vi "Create Data Table.vi"(8 "错误输入（无错误）":errorcluster, 9 "Result":bool[](array[boolean]), 10 "Data":bool[][](array[boolean]), 11 "Data Table":refnum<vi>) -> (0 "错误输出":errorcluster, 3 "Data Table Ref Out":refnum<vi>)   [LabVIEW 2012]
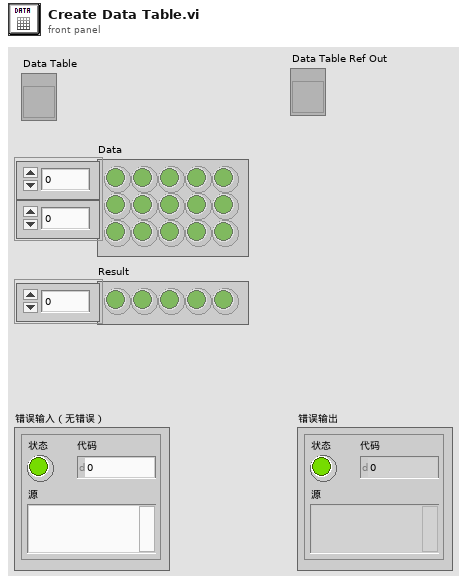
[diagram p1: front panel]
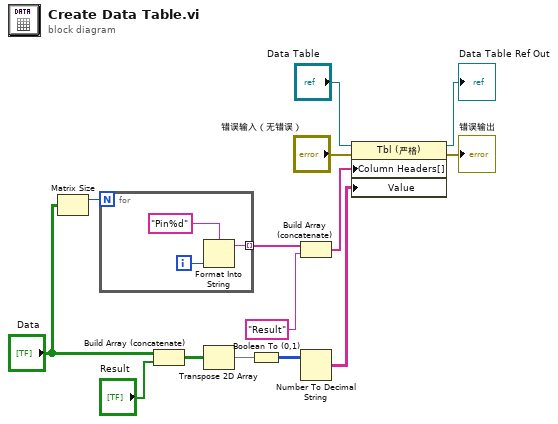
[diagram p0: block diagram]
diagram:
  n1 = Matrix Size(0:"Data") -> (1:w14:i32)  [unwired: 1 out]
  n2 = for {
    N: w14 -> [_]
    tunnel: [w15] -> w12 mode=indexing
    i -> [w17]
    n3 = Format Into String(format string="Pin%d" ("格式字符串"), w17) -> (resulting string=w15:string)  [unwired: 2 in, 1 out]
  }
  n4 = Build Array (concatenate)("Data", "Result") -> (w8:bool[][])
  n5 = Transpose 2D Array(2D array=w8) -> (transposed array=w7:bool[][])
  n6 = Boolean To (0,1)(Boolean=w7) -> (0, 1=w6:i16[][])
  n7 = Build Array (concatenate)(w12, "Result") -> (w11:string[])
  n8 = Number To Decimal String(number=w6) -> (decimal integer string=w1:string[][])  [unwired: 1 in]
  n9 = property on="属性节点" class="Tbl (严格)"(reference="Data Table", error in="错误输入（无错误）", "Column Headers[]"=w11, "Value"=w1) -> (reference out=→"Data Table Ref Out":refnum<vi>, error out=→"错误输出":errorcluster)
